vi "Process 1 Page.vi"() -> ()   [LabVIEW 2019]
uses:
  <vilib>/NI/Current Value Table/Type Defs/Single Tag.ctl
  <vilib>/NI/Current Value Table/Type Defs/Data Types.ctl
  <vilib>/NI/STM/TCP/Read Meta Data (TCP Ref).vi
  <vilib>/NI/STM/TCP/Get Connection Reference (TCP).vi
  <vilib>/NI/AMC/Read Termination Message.vi
  <vilib>/NI/AMC/Create Single Message.vi
  <vilib>/NI/AMC/Update Message Routing Info.vi
  <vilib>/NI/STM/TCP/Read Meta Data (TCP Clst).vi
  <vilib>/NI/AMC/Globals.vi
  <vilib>/NI/STM/TCP/Write Message (TCP).vi
  <vilib>/NI/AMC/Send Message.vi
  <vilib>/NI/AMC/AMC.lvlib
  <vilib>/NI/STM/NI STM.lvlib
  <vilib>/NI/Current Value Table/Current Value Table.lvlib
panel:
  out "Boolean 5":bool
  out "Pressure (kPa)":dbl(knob) scale=0.0..150.0
  out "RPM":dbl(knob) scale=0.0..3500.0
  out "DI Flow Rate":dbl(knob) scale=0.0..75.0
  in  "Oxide grams to Add 1":dbl=2.0 caption="Oxide grams to Add" min=-1000.0 max=1000.0 step=0.1
  in  "Dose Extra Oxide 1":bool caption="Dose Extra Oxide"
  in  "Flow to Oxide 1":dbl=2.0 caption="Flow to Oxide" min=2.0 max=12.0 step=0.1
  in  "Enable Oxide System 1":bool caption="Enable Oxide System"
  out "SG":dbl format="%.4g"
  in  "Bath SG":dbl=1.8 min=0.9 max=1.8 step=0.0025 format="%.4g"
  out "Recirc Elbow":bool
  out "Di Add Pipe":bool
  out "Di Water Elbow":bool
  out "Liters DI Added 1":dbl caption="Liters DI Added" format="%.1f"
  in  "T Setpoint 1":dbl=15.0 caption="T Setpoint" min=15.0 max=28.0 step=0.5
  in  "Enable T Control 1":bool caption="Enable T Control"
  in  "DI Add Volume 1":dbl caption="DI Add Volume" min=0.0 max=500.0 step=0.25
  in  "Add DI water 1":bool caption="Add DI Water"
  in  "Drain System to Tree 1":bool caption="Drain System to Tree"
  in  "Enable Main Pump":bool
  out "FlowToOxSys 1":dbl(slide) caption="Flow To Oxide Sys" scale=0.0..12.0 scale format="%.1f"
  out "Oxide Pump":bool
  out "Chilled Water Injection 1":u8(slide) caption="Chilled Water Injection" scale=0.0..100.0
  out "Tempered Water Injection 1":u8(slide) caption="Tempered Water Injection" scale=0.0..100.0
  out "Process 1 Supply":bool
  out "Sump Return":bool
  out "PipeFromPmp":bool
  out "Plating Tanks In Use South PE":bool
  out "Oxide Left To Dose":dbl format="%#.1f"
  out "OxideDose Indicate 1":bool caption="Oxide Dosing"
  out "T °C 1":dbl(slide) caption="T °C" scale=0.0..30.0
  out "Proc4MainPumpInd 2":bool
  out "Tank 1":dbl(slide) caption="Tank" scale=0.0..1000.0
  out "Run Enabled":bool
  in  "Dosing":bool
  in  "Mixing Tank":bool
  in  "Process 3":bool
  in  "Process 2":bool
  in  "Process 1":bool
  out "status":string
  in  "Home Btn":bool
  in  "Facilities Btn":bool
  # "T 341"
  # "@"
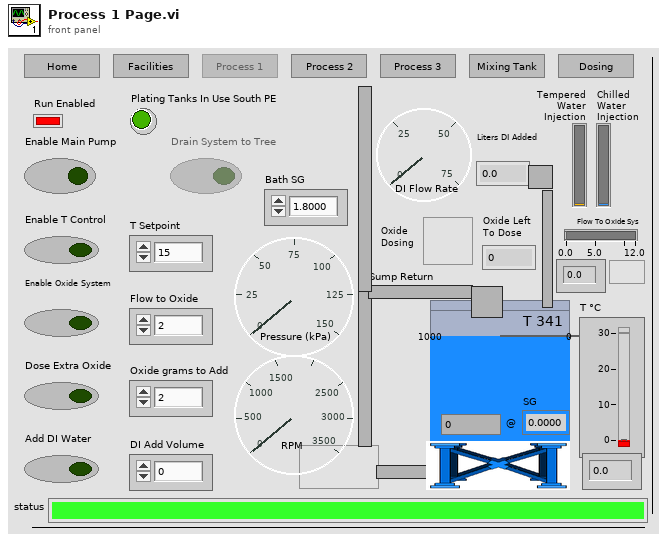
[diagram p1: front panel]
types:
  T1 = typedef "Current Value Table.lvlib/Single Tag.ctl" = cluster{"Data Type":T2, "Name":string, "Value":string, "Description":string}
  T2 = typedef "Current Value Table.lvlib/Data Types.ctl" = enum16{"Double", "Single", "I64", "I32", "I16", "I8", "U64", "U32", "U16", "U8", "String", "Boolean", "Array of U8", "Array of U16", "Array of U32", "Array of U64", "Array of I64", "Array of I32", "Array of I16", "Array of I8", "Array of Double", "Array of Single", "Array of Boolean", "Array of String"}
  T3 = typedef "AMC.lvlib/Message Queue.ctl" = refnum<queue>
  T4 = typedef "NI STM.lvlib/TCP Connection Info.ctl" = cluster{"connection ID":refnum<k5>, "meta data":T5[]}
  T5 = typedef "NI STM.lvlib/MetaDataElement.ctl" = string
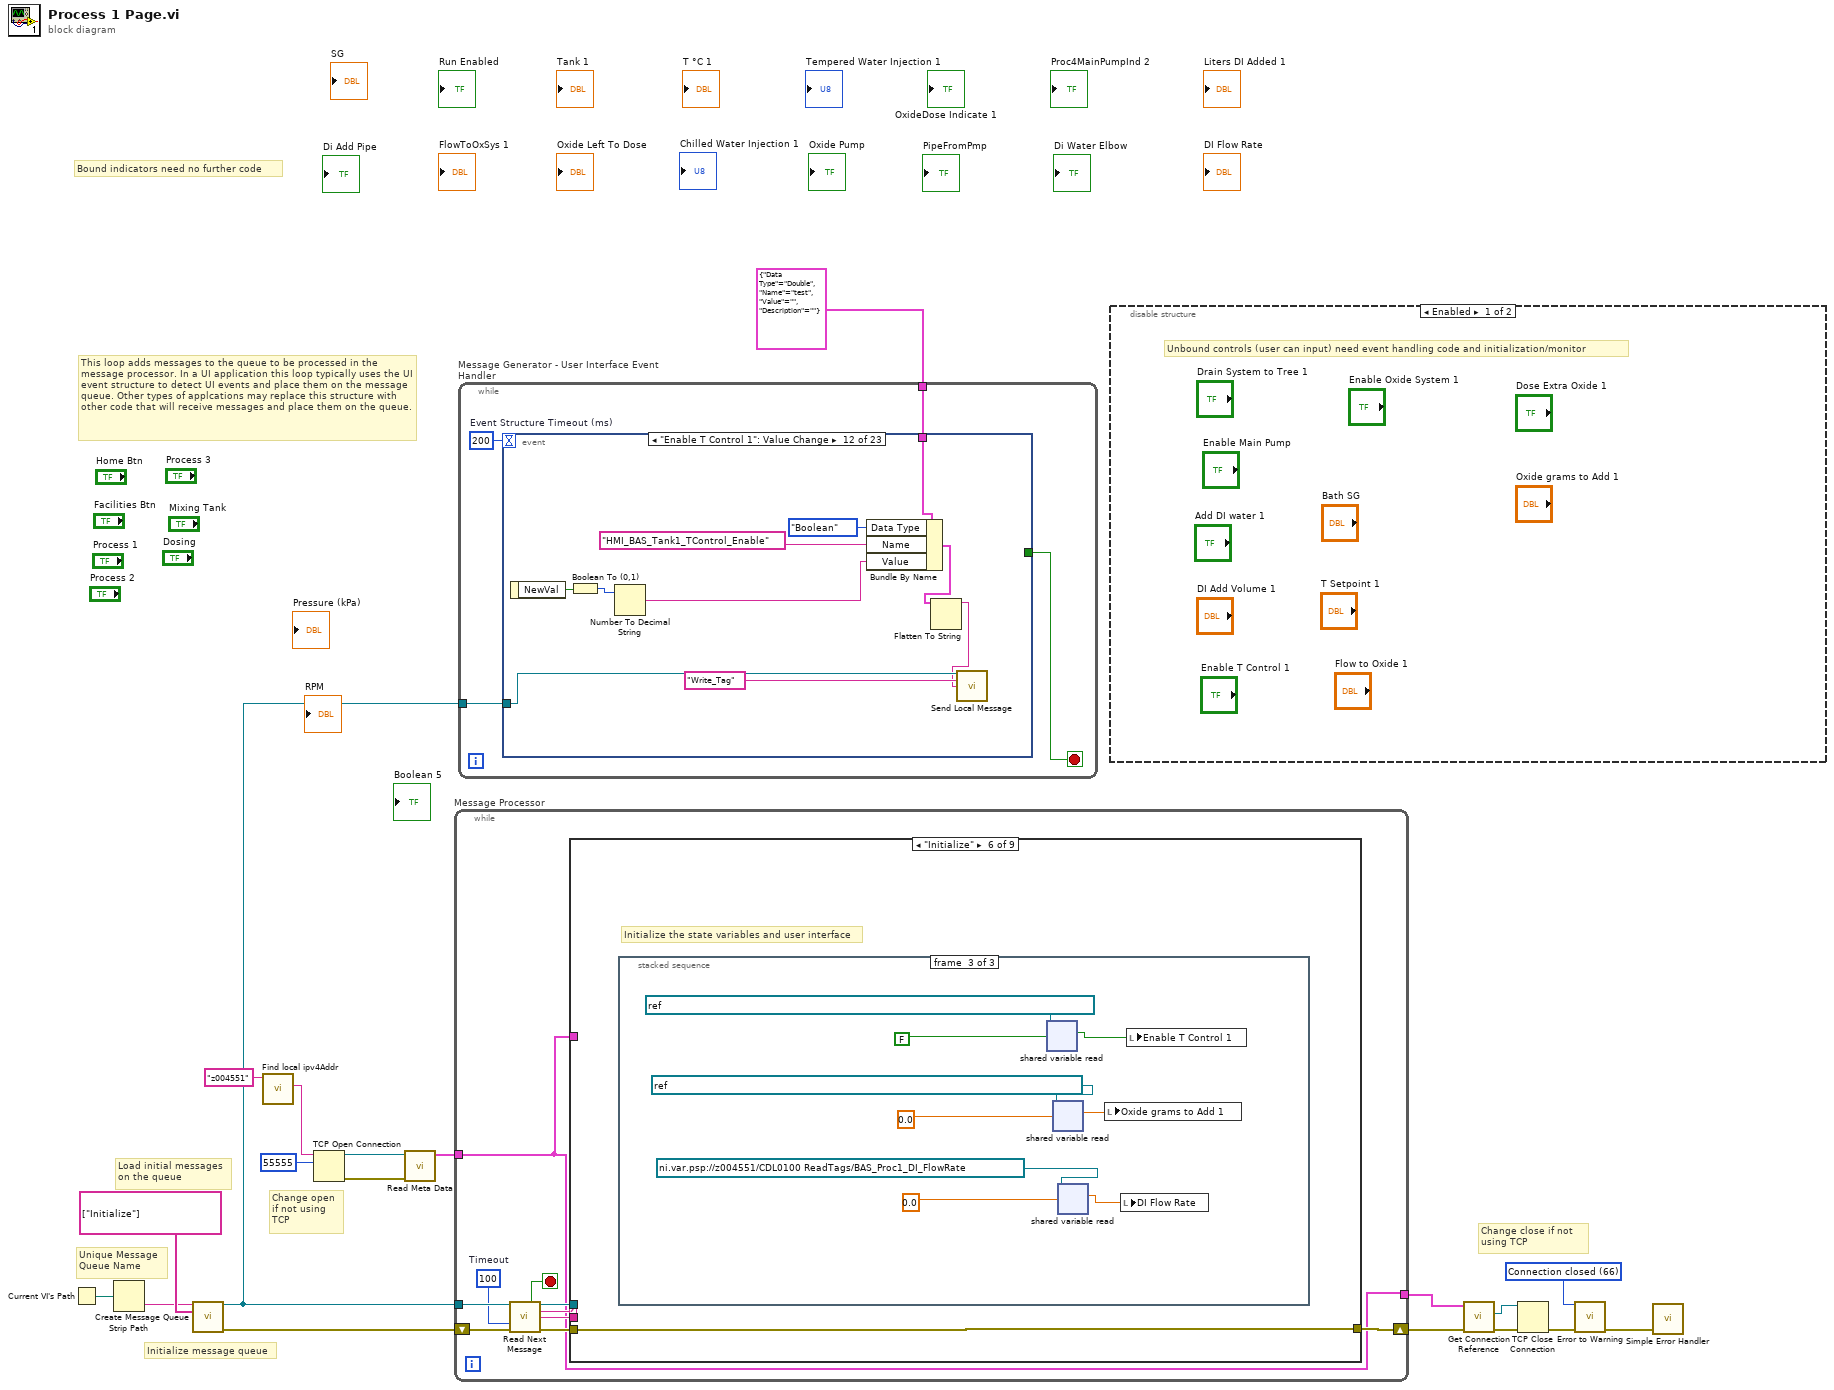
[diagram p0: block diagram]
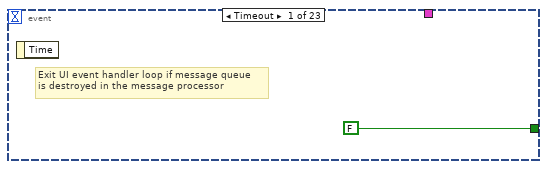
[diagram p3: hidden frame]
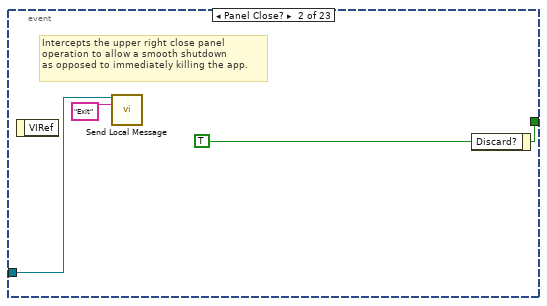
[diagram p4: hidden frame]
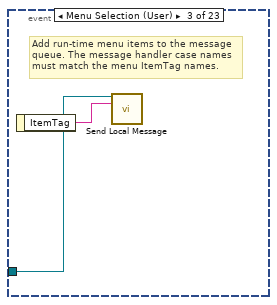
[diagram p5: hidden frame]
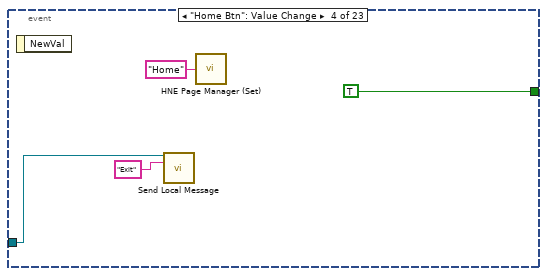
[diagram p6: hidden frame]
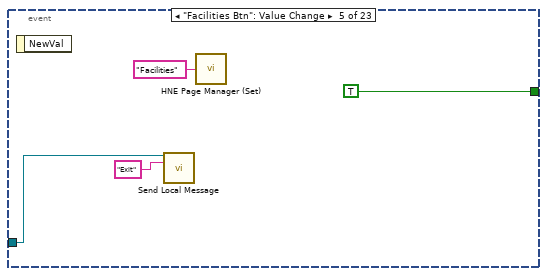
[diagram p7: hidden frame]
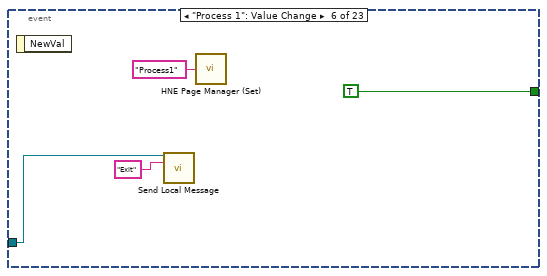
[diagram p8: hidden frame]
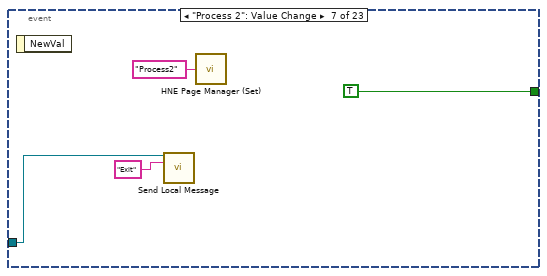
[diagram p9: hidden frame]
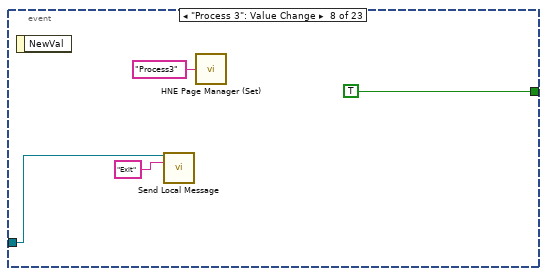
[diagram p10: hidden frame]
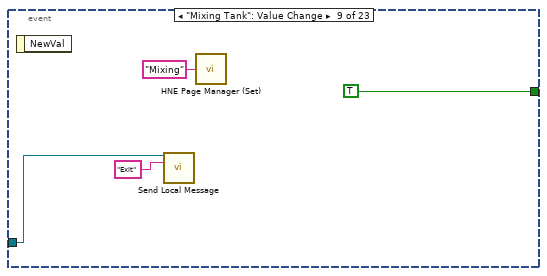
[diagram p11: hidden frame]
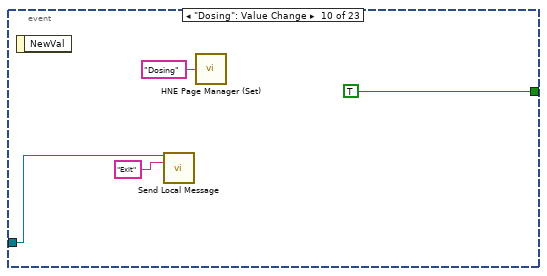
[diagram p12: hidden frame]
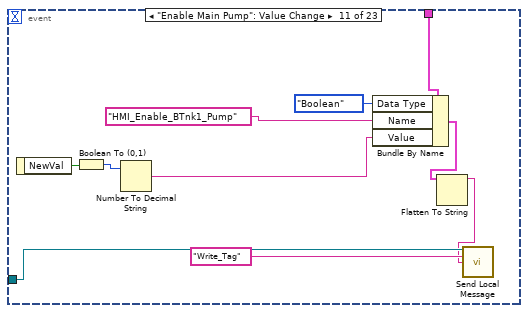
[diagram p13: hidden frame]
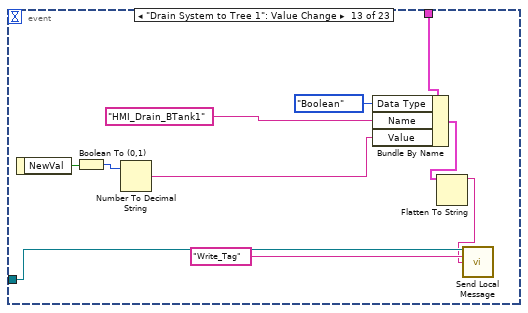
[diagram p14: hidden frame]
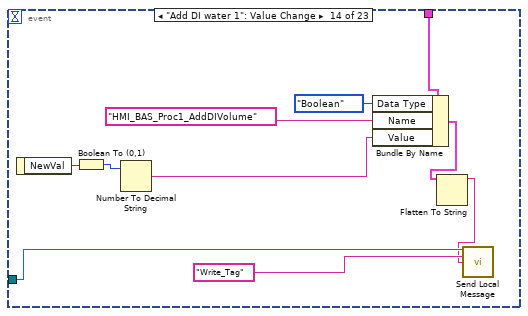
[diagram p15: hidden frame]
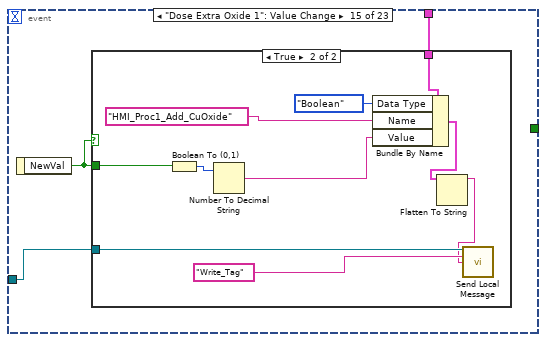
[diagram p16: hidden frame]
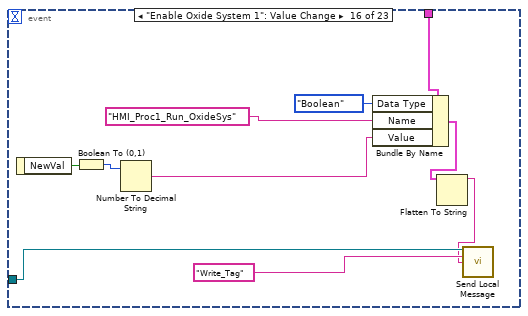
[diagram p18: hidden frame]
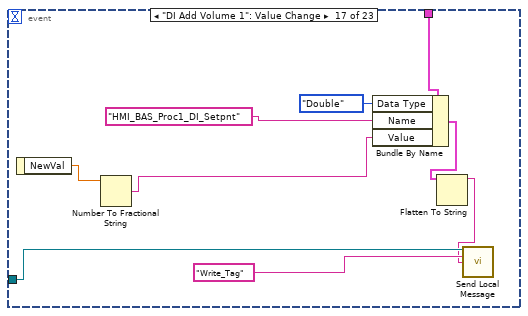
[diagram p19: hidden frame]
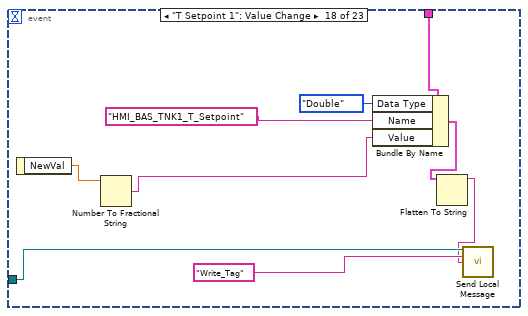
[diagram p20: hidden frame]
diagram:
  w8 = 66 items=["No Error", "Argument Error", "Memory Full", "Out of Zone", "End of File", "File Already Open", "Generic File IO Error", "File Not Found", "File Permission Error", "Disk Full", "Duplicate Path", "Too Many Files Open", "Not Enabled", "Resource File Not Found", "Cannot Add Resource", "Resource Not Found", "Image Not Found", "Image Memory Error", "Pen Does Not Exist", "Config Bad Type", "Config Token Not Found", "Config Parse Error", "Config Memory Error", "Bad External Code Format", "Bad External Code Offset", "External Code Not Present", "Null Window", "Destroy Window Mixup", "Null Menu", "Print Aborted", "Bad Print Record", "Print Driver Error", "Windows Error During Print", "Memory Error During Print", "Print Dialog Error", "Generic Print Error", "Invalid Device Refnum", "Device Not Found", "Device Parameter Error", "Device Unit Error", "Can't Open Device", "Device Call Aborted", "Generic Error", "Cancelled By User", "Object ID Too Low", "Object ID Too High", "Object Not In Heap", "Unknown Heap", "Bad DefProc ID", "DefProc Not In Table", "Message Out Of Range", "Null Method", "Unknown Message", "Manager Call Not Supported", "Bad address", "Connection In progress", "Connection timed out", "Connection is already in progress", "Network attribute not supported", "Network error", "Address in use", "System out of memory", "Connection aborted", "Connection refused", "Connection is not connected", "Connection is already connected", "Connection closed", "Initialize error (interapplication manager)", "Bad occurrence", "Wait on unbound occurrence handler", "Occurrence queue overflow", "Bad path", "Semaphore not signaled", "Unrecognized type (interapplication manager)"] ("1st Error to Convert")
  # "Bound indicators need no further code"
  # "Change close if not using TCP"
  # "Change open if not using TCP"
  # "This loop adds messages to the queue to be processed in the message processor. In a UI application this loop typically uses the UI event structure to detect UI events and place them on the message queue. Other types of applcations may replace this structure with other code that will receive messages and place them on the queue."
  # "Initialize message queue"
  # "Unique Message\nQueue Name"
  # "Load initial messages\non the queue"
  n1 = Current VI's Path() -> (path=w15:path)
  n2 = Strip Path(path=w15) -> (name=w18:string)  [unwired: 1 out]
  n3 = call <vilib>:"Create Message Queue.vi"("message queue name"=w18, "initial message names"=string[] ["Initialize"]) -> ("message queue out"=w17:T3, "error out"=w16:errorcluster)  [unwired: 12 in]
  n4 = call "Find local ipv4Addr.vi"("MachineToFind"="z004551") -> ("name"=w11:string)  [unwired: 9 in, 1 out]
  n5 = TCP Open Connection(address=w11, remote port or service name=u16 55555 ("remote port")) -> (connection ID=w13:refnum<k5>, error out=w12:errorcluster)  [unwired: 1 in, 2 out]
  n6 = call-poly <vilib>:"Read Meta Data.vi"("error in"=w12, "connection ID"=w13) -> ("connection info out"=w3:T4)  [unwired: 7 in, 2 out]
  n7 = while "Message Processor" {
    shift-left: w16 -> [w25]
    shift-right: [w29] -> w4
    tunnel: w17 -> [w26]
    tunnel: [w20] -> w2
    tunnel: w3 -> [w20]
    stop <- w28 stop-if-true
    w21 = 100  # Timeout
    n8 = call <vilib>:"Read Next Message.vi"("message queue in"=w26, "timeout (1 ms)"=w21, "error in"=w25) -> ("exit process?"=w28:bool, "message queue out"=w27:T3, "message name"=w23:string, "message value"=w22:string, "error out"=w24:errorcluster)  [unwired: 5 in, 3 out]
    n9 = case shown="\"Initialize\"" w23 {
      selector: w23 -> [_ _ w69 _ _ _ _ _ _]
      tunnel: w27 -> [_ _ _ _ _ _ w109 _ _]
      tunnel: w24 -> [w30 w32 w70 w71 w73 w74 w110 w112 w114]
      tunnel: [w30 w32 w70 errorcluster {"status"=FALSE, "code"=0, "source"=""} ("error out") w73 w74 w108 w112 w113] -> w29
      tunnel: w22 -> [_ _ _ _ _ _ _ _ w115]
      tunnel: w20 -> [_ _ _ _ _ _ _ _ w116]
      frame "---------- Framework Operations ----------" {
        # "Dummy case to add a seperator in the Case Structure menu"
      }
      frame "", "Idle" {
        # "Idle Case - this case is called after a Timeout on the Get Next Message from Queue VI, if no new messages are present on the queue. This case can be used for housekeeping tasks such as updating the UI."
        n10 = stacked-sequence {
          frame #0 {
            # "Other HMI changed state - align"
            n11 = shared-variable-read(refnum<k21> "ni.var.psp://z004551/CDL0100 ReadWriteTags/HMI_Enable_BTnk1_Pump" ("shared variable refnum in"), FALSE ("data type")) -> (w33:bool)  [unwired: 1 in, 3 out]
            n12 = shared-variable-read(refnum<k21> "ni.var.psp://z004551/CDL0100 ReadWriteTags/HMI_Tank2_Enable" ("shared variable refnum in"), FALSE) -> (w41:bool)  [unwired: 1 in, 3 out]
            n13 = shared-variable-read(refnum<k21> "ni.var.psp://z004551/CDL0100 ReadWriteTags/HMI_Tank1_Enable" ("shared variable refnum in"), FALSE) -> (w36:bool)  [unwired: 1 in, 3 out]
            n14 = Or(x=w36, y=w41) -> (x .or. y?=→"Plating Tanks In Use South PE":bool)
            n15 = call <userlib>:"Boolean Trigger__ogtk.vi"("Boolean Input"=w33) -> ("Rising Edge"=w39:bool, "Falling Edge"=w38:bool)  [unwired: 1 in]
            n16 = Or(x=w39, y=w38) -> (x .or. y?=w37:bool)
            n17 = case shown="True" w37 {
              tunnel: w33 -> [_ w46]
              frame False {
              }
              frame True {
                n18 = local write "Enable Main Pump"(w46) -> ()
              }
            }
          }
          frame #1 {
            n19 = shared-variable-read(refnum<k21> "ni.var.psp://z004551/CDL0100 ReadTags/IO_Bas_Tnk1_3Way_At_Open" ("shared variable refnum in"), FALSE) -> (w49:bool)  [unwired: 1 in, 3 out]
            n20 = shared-variable-read(refnum<k21> "ni.var.psp://z004551/CDL0100 ReadTags/IO_Bas_Tnk1_3Way_At_Recirc" ("shared variable refnum in"), FALSE) -> (w48:bool)  [unwired: 1 in, 3 out]
            n21 = shared-variable-read(refnum<k21> "ni.var.psp://z004551/CDL0100 ReadTags/IO_Bas_Tnk1_3Way_At_Closed" ("shared variable refnum in"), FALSE) -> (w51:bool)  [unwired: 1 in, 3 out]
            n22 = Or(x=w51, y=w49) -> (x .or. y?=→"Process 1 Supply":bool)
            n23 = Or(x=w49, y=w48) -> (x .or. y?=→"Sump Return" →"Recirc Elbow":bool)
          }
          frame #2 {
            n24 = shared-variable-read(refnum<k21> "ni.var.psp://z004551/CDL0100 ReadWriteTags/HMI_BAS_Proc1_AddDIVolume" ("shared variable refnum in"), FALSE) -> (w59:bool)  [unwired: 1 in, 3 out]
            n25 = call <userlib>:"Boolean Trigger__ogtk.vi"("Boolean Input"=w59) -> ("Falling Edge"=w58:bool)  [unwired: 1 in, 1 out]
            n26 = case shown="True" w58 {
              frame False {
              }
              frame True {
                n27 = local write "Add DI water 1"(FALSE) -> ()
              }
            }
          }
          frame #3 {
            n28 = control-ref of="Enable Main Pump"() -> (w63:refnum<vi>)
            n29 = control-ref of="Drain System to Tree 1"() -> (w65:refnum<vi>)
            n30 = call "GrayOutButtonFromPSPVar.vi"("shared variable refnum in"=refnum<k21> "ni.var.psp://z004551/CDL0100 ReadWriteTags/HMI_Drain_BTank1", "Boolean in"=w63) -> ()  [unwired: 10 in]
            n31 = call "GrayOutButtonFromPSPVar.vi"("shared variable refnum in"=refnum<k21> "ni.var.psp://z004551/CDL0100 ReadWriteTags/HMI_Enable_BTnk1_Pump", "Boolean in"=w65) -> ()  [unwired: 10 in]
          }
        }
        n32 = control-ref of="status"() -> (w31:refnum<vi>)
        n33 = call <userlib>:"TAE Format Alarm Ticker.vi"("Alarm Ticker Ref"=w31) -> ()  [unwired: 15 in]
      }
      frame "Missing Message Handler", Default {
        # "Call this case if a message is received that is not handled \nby any other case. Typically this is a programming error\nas a result of a typo or unhandled message/missing message handler."
        n34 = Format Into String(format string="DevError: Missing message handler for '%s\" message." ("message"), w69) -> (resulting string=w67:string)  [unwired: 2 in, 1 out]
        n35 = One Button Dialog(message=w67) -> ()  [unwired: 2 out]
      }
      frame "Error" {
        # "General Error Case - this case is called if an error is passed using the error cluster below. Typically most new errors should be handed in each individual case and not passed in the rror cluster. If necessary a custom error handler case should be added and called from other cases."
        n36 = call <vilib>:"Simple Error Handler.vi"("error in (no error)"=w71) -> ()  [unwired: 1 in, 8 out]
      }
      frame "---------- Generic Operations ----------" {
        # "Dummy case to add a seperator in the Case Structure menu"
      }
      frame "Initialize" {
        # "Initialize the state variables and user interface"
        n37 = stacked-sequence {
          frame #0 {
            n38 = shared-variable-read(refnum<k21> "ni.var.psp://z004551/CDL0100 ReadWriteTags/HMI_Drain_BTank1" ("shared variable refnum in"), FALSE) -> (w81:bool)  [unwired: 1 in, 3 out]
            n39 = shared-variable-read(refnum<k21> "ni.var.psp://z004551/CDL0100 ReadWriteTags/HMI_BAS_Proc1_AddDIVolume" ("shared variable refnum in"), FALSE) -> (w78:bool)  [unwired: 1 in, 3 out]
            n40 = shared-variable-read(refnum<k21> "ni.var.psp://z004551/CDL0100 ReadWriteTags/HMI_Enable_BTnk1_Pump" ("shared variable refnum in"), FALSE) -> (w84:bool)  [unwired: 1 in, 3 out]
            n41 = shared-variable-read(refnum<k21> "ni.var.psp://z004551/CDL0100 ReadWriteTags/HMI_BAS_Proc1_DI_Setpnt" ("shared variable refnum in"), 0.0) -> (w75:dbl)  [unwired: 1 in, 3 out]
            n42 = local write "Drain System to Tree 1"(w81) -> ()
            n43 = local write "Add DI water 1"(w78) -> ()
            n44 = local write "Enable Main Pump"(w84) -> ()
            n45 = local write "DI Add Volume 1"(w75) -> ()
          }
          frame #1 {
            n46 = shared-variable-read(refnum<k21> "ni.var.psp://z004551/CDL0100 ReadWriteTags/HMI_Proc1_Run_OxideSys" ("shared variable refnum in"), FALSE) -> (w87:bool)  [unwired: 1 in, 3 out]
            n47 = shared-variable-read(refnum<k21> "ni.var.psp://z004551/CDL0100 ReadWriteTags/HMI_Proc1_OxFlow_SetPnt" ("shared variable refnum in"), 0.0) -> (w90:dbl)  [unwired: 1 in, 3 out]
            n48 = shared-variable-read(refnum<k21> "ni.var.psp://z004551/CDL0100 ReadWriteTags/HMI_BAS_TNK1_T_Setpoint" ("shared variable refnum in"), 0.0) -> (w93:dbl)  [unwired: 1 in, 3 out]
            n49 = shared-variable-read(refnum<k21> "ni.var.psp://z004551/CDL0100 ReadWriteTags/HMI_BAS_Proc1_Tank_SG" ("shared variable refnum in"), 0.0) -> (w96:dbl)  [unwired: 1 in, 3 out]
            n50 = local write "Enable Oxide System 1"(w87) -> ()
            n51 = local write "T Setpoint 1"(w93) -> ()
            n52 = local write "Flow to Oxide 1"(w90) -> ()
            n53 = local write "Bath SG"(w96) -> ()
          }
          frame #2 {
            n54 = shared-variable-read(refnum<k21> "ni.var.psp://z004551/CDL0100 ReadWriteTags/HMI_BAS_Tank1_TControl_Enable" ("shared variable refnum in"), FALSE) -> (w105:bool)  [unwired: 1 in, 3 out]
            n55 = shared-variable-read(refnum<k21> "ni.var.psp://z004551/CDL0100 ReadWriteTags/HMI_Proc1_CuOxideAddAmnt" ("shared variable refnum in"), 0.0) -> (w102:dbl)  [unwired: 1 in, 3 out]
            n56 = shared-variable-read(refnum<k21> "ni.var.psp://z004551/CDL0100 ReadTags/BAS_Proc1_DI_FlowRate" ("shared variable refnum in"), 0.0) -> (w99:dbl)  [unwired: 1 in, 3 out]
            n57 = local write "Oxide grams to Add 1"(w102) -> ()
            n58 = local write "DI Flow Rate"(w99) -> ()
            n59 = local write "Enable T Control 1"(w105) -> ()
          }
        }
      }
      frame "Exit" {
        # "Destroy message queue >> this will halt the UI event handler loop"
        # "Stop the VI\n>> Perform any cleanup tasks in this message case.\n>> Clear display before closing."
        n60 = call <vilib>:"Destroy Message Queue.vi"("message queue in"=w109, "error in"=w110) -> ("error out"=w108:errorcluster)  [unwired: 11 in, 2 out]
        n61 = local write "status"("" ("Status")) -> ()
      }
      frame "---------- Application Operations ----------" {
        # "Dummy case to add a seperator in the Case Structure menu"
      }
      frame "Write_Tag" {
        n62 = call-poly <vilib>:"Write Message.vi"("error in"=w114, "data"=w115, "name"="WriteTag", "connection info in"=w116) -> ("error out"=w113:errorcluster)  [unwired: 6 in, 1 out]
      }
    }
  }
  n63 = while "Message Generator - User Interface Event Handler" {
    tunnel: w17 -> [w119]
    tunnel: T1 {"Data Type"=enum."Double", "Name"="test", "Value"="", "Description"=""} ("Tag") -> [w118]
    stop <- w120 stop-if-true
    w121 = 200  # Event Structure Timeout (ms)
    n64 = event shown="[11] \"Enable T Control 1\": Value Change" {
      selector: _ -> [_ _ _ _ _ _ _ _ _ _ _ _ _ _ _ _ _ _ _ _ _ _ _]
      dyn-events: _ -> [_ _ _ _ _ _ _ _ _ _ _ _ _ _ _ _ _ _ _ _ _ _ _]
      timeout: w121 -> [_ _ _ _ _ _ _ _ _ _ _ _ _ _ _ _ _ _ _ _ _ _ _]
      tunnel: [FALSE ("Discard?") w125 _ TRUE ("Discard?") TRUE ("Discard?") TRUE ("Discard?") TRUE ("Discard?") TRUE ("Discard?") TRUE ("Discard?") TRUE ("Discard?") _ _ _ _ _ _ _ _ _ _ _ _ _] -> w120
      tunnel: w119 -> [_ w123 w126 w128 w132 w136 w140 w144 w148 w152 w158 w168 w178 w188 w197 w211 w223 w232 w241 w250 w259 _ _]
      tunnel: w118 -> [_ _ _ _ _ _ _ _ _ _ w163 w173 w183 w193 w198 w216 w227 w236 w245 w254 w263 _ _]
      event Timeout {
        # "Exit UI event handler loop if message queue\nis destroyed in the message processor"
        n65 = event-data() -> ()  [unwired: 2 out]
      }
      event Panel Close? {
        w125 = TRUE ("Discard?")
        # "Intercepts the upper right close panel\noperation to allow a smooth shutdown\nas opposed to immediately killing the app."
        n66 = event-data() -> ()  [unwired: 2 out]
        n67 = call <vilib>:"Send Local Message.vi"("message queue in"=w123, "message name"="Exit") -> ()  [unwired: 11 in, 3 out]
        n68 = event-data("Discard?"=w125) -> ()  [unwired: 1 in, 1 out]
      }
      event Menu Selection (User) {
        # "Add run-time menu items to the message\nqueue. The message handler case names must match the menu ItemTag names."
        n69 = event-data() -> ("ItemTag"=w127:string)  [unwired: 1 out]
        n70 = call <vilib>:"Send Local Message.vi"("message queue in"=w126, "message name"=w127) -> ()  [unwired: 11 in, 3 out]
      }
      event "Home Btn": Value Change {
        n71 = event-data() -> ()  [unwired: 2 out]
        n72 = call <vilib>:"Send Local Message.vi"("message queue in"=w128, "message name"="Exit") -> ()  [unwired: 11 in, 3 out]
        n73 = call <userlib>:"HNE Page Manager (Set).vi"("Next Page"="Home") -> ()  [unwired: 4 in, 1 out]
      }
      event "Facilities Btn": Value Change {
        n74 = event-data() -> ()  [unwired: 2 out]
        n75 = call <vilib>:"Send Local Message.vi"("message queue in"=w132, "message name"="Exit") -> ()  [unwired: 11 in, 3 out]
        n76 = call <userlib>:"HNE Page Manager (Set).vi"("Next Page"="Facilities") -> ()  [unwired: 4 in, 1 out]
      }
      event "Process 1": Value Change {
        n77 = event-data() -> ()  [unwired: 2 out]
        n78 = call <vilib>:"Send Local Message.vi"("message queue in"=w136, "message name"="Exit") -> ()  [unwired: 11 in, 3 out]
        n79 = call <userlib>:"HNE Page Manager (Set).vi"("Next Page"="Process1") -> ()  [unwired: 4 in, 1 out]
      }
      event "Process 2": Value Change {
        n80 = event-data() -> ()  [unwired: 2 out]
        n81 = call <vilib>:"Send Local Message.vi"("message queue in"=w140, "message name"="Exit") -> ()  [unwired: 11 in, 3 out]
        n82 = call <userlib>:"HNE Page Manager (Set).vi"("Next Page"="Process2") -> ()  [unwired: 4 in, 1 out]
      }
      event "Process 3": Value Change {
        n83 = event-data() -> ()  [unwired: 2 out]
        n84 = call <vilib>:"Send Local Message.vi"("message queue in"=w144, "message name"="Exit") -> ()  [unwired: 11 in, 3 out]
        n85 = call <userlib>:"HNE Page Manager (Set).vi"("Next Page"="Process3") -> ()  [unwired: 4 in, 1 out]
      }
      event "Mixing Tank": Value Change {
        n86 = event-data() -> ()  [unwired: 2 out]
        n87 = call <vilib>:"Send Local Message.vi"("message queue in"=w148, "message name"="Exit") -> ()  [unwired: 11 in, 3 out]
        n88 = call <userlib>:"HNE Page Manager (Set).vi"("Next Page"="Mixing") -> ()  [unwired: 4 in, 1 out]
      }
      event "Dosing": Value Change {
        n89 = event-data() -> ()  [unwired: 2 out]
        n90 = call <vilib>:"Send Local Message.vi"("message queue in"=w152, "message name"="Exit") -> ()  [unwired: 11 in, 3 out]
        n91 = call <userlib>:"HNE Page Manager (Set).vi"("Next Page"="Dosing") -> ()  [unwired: 4 in, 1 out]
      }
      event "Enable Main Pump": Value Change {
        n92 = event-data() -> ("NewVal"=w165:bool)  [unwired: 1 out]
        n93 = Boolean To (0,1)(Boolean=w165) -> (0, 1=w164:i16)
        n94 = Number To Decimal String(number=w164) -> (decimal integer string=w160:string)  [unwired: 1 in]
        n95 = Bundle By Name(cluster=w163, "Data Type"=Data_Types."Boolean", "Name"="HMI_Enable_BTnk1_Pump", "Value"=w160) -> (w159:T1)
        n96 = Flatten To String(anything=w159) -> (data string=w156:string)  [unwired: 3 in, 2 out]
        n97 = call <vilib>:"Send Local Message.vi"("message queue in"=w158, "message name"="Write_Tag", "message value"=w156) -> ()  [unwired: 10 in, 3 out]
      }
      event "Enable T Control 1": Value Change {
        n98 = event-data() -> ("NewVal"=w175:bool)  [unwired: 1 out]
        n99 = Boolean To (0,1)(Boolean=w175) -> (0, 1=w174:i16)
        n100 = Number To Decimal String(number=w174) -> (decimal integer string=w170:string)  [unwired: 1 in]
        n101 = Bundle By Name(cluster=w173, "Data Type"=Data_Types."Boolean", "Name"="HMI_BAS_Tank1_TControl_Enable", "Value"=w170) -> (w169:T1)
        n102 = Flatten To String(anything=w169) -> (data string=w166:string)  [unwired: 3 in, 2 out]
        n103 = call <vilib>:"Send Local Message.vi"("message queue in"=w168, "message name"="Write_Tag", "message value"=w166) -> ()  [unwired: 10 in, 3 out]
      }
      event "Drain System to Tree 1": Value Change {
        n104 = event-data() -> ("NewVal"=w185:bool)  [unwired: 1 out]
        n105 = Boolean To (0,1)(Boolean=w185) -> (0, 1=w184:i16)
        n106 = Number To Decimal String(number=w184) -> (decimal integer string=w180:string)  [unwired: 1 in]
        n107 = Bundle By Name(cluster=w183, "Data Type"=Data_Types."Boolean", "Name"="HMI_Drain_BTank1", "Value"=w180) -> (w179:T1)
        n108 = Flatten To String(anything=w179) -> (data string=w176:string)  [unwired: 3 in, 2 out]
        n109 = call <vilib>:"Send Local Message.vi"("message queue in"=w178, "message name"="Write_Tag", "message value"=w176) -> ()  [unwired: 10 in, 3 out]
      }
      event "Add DI water 1": Value Change {
        n110 = event-data() -> ("NewVal"=w195:bool)  [unwired: 1 out]
        n111 = Boolean To (0,1)(Boolean=w195) -> (0, 1=w194:i16)
        n112 = Number To Decimal String(number=w194) -> (decimal integer string=w190:string)  [unwired: 1 in]
        n113 = Bundle By Name(cluster=w193, "Data Type"=Data_Types."Boolean", "Name"="HMI_BAS_Proc1_AddDIVolume", "Value"=w190) -> (w189:T1)
        n114 = Flatten To String(anything=w189) -> (data string=w186:string)  [unwired: 3 in, 2 out]
        n115 = call <vilib>:"Send Local Message.vi"("message queue in"=w188, "message name"="Write_Tag", "message value"=w186) -> ()  [unwired: 10 in, 3 out]
      }
      event "Dose Extra Oxide 1": Value Change {
        n116 = event-data() -> ("NewVal"=w196:bool)  [unwired: 1 out]
        n117 = case shown="True" w196 {
          tunnel: w196 -> [_ w208]
          tunnel: w198 -> [_ w206]
          tunnel: w197 -> [_ w201]
          frame False {
          }
          frame True {
            n118 = Boolean To (0,1)(Boolean=w208) -> (0, 1=w207:i16)
            n119 = Number To Decimal String(number=w207) -> (decimal integer string=w203:string)  [unwired: 1 in]
            n120 = Bundle By Name(cluster=w206, "Data Type"=Data_Types."Boolean", "Name"="HMI_Proc1_Add_CuOxide", "Value"=w203) -> (w202:T1)
            n121 = Flatten To String(anything=w202) -> (data string=w199:string)  [unwired: 3 in, 2 out]
            n122 = call <vilib>:"Send Local Message.vi"("message queue in"=w201, "message name"="Write_Tag", "message value"=w199) -> ()  [unwired: 10 in, 3 out]
          }
        }
      }
      event "Enable Oxide System 1": Value Change {
        n123 = event-data() -> ("NewVal"=w218:bool)  [unwired: 1 out]
        n124 = Boolean To (0,1)(Boolean=w218) -> (0, 1=w217:i16)
        n125 = Number To Decimal String(number=w217) -> (decimal integer string=w213:string)  [unwired: 1 in]
        n126 = Bundle By Name(cluster=w216, "Data Type"=Data_Types."Boolean", "Name"="HMI_Proc1_Run_OxideSys", "Value"=w213) -> (w212:T1)
        n127 = Flatten To String(anything=w212) -> (data string=w209:string)  [unwired: 3 in, 2 out]
        n128 = call <vilib>:"Send Local Message.vi"("message queue in"=w211, "message name"="Write_Tag", "message value"=w209) -> ()  [unwired: 10 in, 3 out]
      }
      event "DI Add Volume 1": Value Change {
        n129 = event-data() -> ("NewVal"=w220:dbl)  [unwired: 1 out]
        n130 = Number To Fractional String(number=w220) -> (F-format string=w219:string)  [unwired: 3 in]
        n131 = Bundle By Name(cluster=w227, "Data Type"=Data_Types."Double", "Name"="HMI_BAS_Proc1_DI_Setpnt", "Value"=w219) -> (w224:T1)
        n132 = Flatten To String(anything=w224) -> (data string=w221:string)  [unwired: 3 in, 2 out]
        n133 = call <vilib>:"Send Local Message.vi"("message queue in"=w223, "message name"="Write_Tag", "message value"=w221) -> ()  [unwired: 10 in, 3 out]
      }
      event "T Setpoint 1": Value Change {
        n134 = event-data() -> ("NewVal"=w229:dbl)  [unwired: 1 out]
        n135 = Number To Fractional String(number=w229) -> (F-format string=w228:string)  [unwired: 3 in]
        n136 = Bundle By Name(cluster=w236, "Data Type"=Data_Types."Double", "Name"="HMI_BAS_TNK1_T_Setpoint", "Value"=w228) -> (w233:T1)
        n137 = Flatten To String(anything=w233) -> (data string=w230:string)  [unwired: 3 in, 2 out]
        n138 = call <vilib>:"Send Local Message.vi"("message queue in"=w232, "message name"="Write_Tag", "message value"=w230) -> ()  [unwired: 10 in, 3 out]
      }
      event "Bath SG": Value Change {
        n139 = event-data() -> ("NewVal"=w238:dbl)  [unwired: 1 out]
        n140 = Number To Fractional String(number=w238) -> (F-format string=w237:string)  [unwired: 3 in]
        n141 = Bundle By Name(cluster=w245, "Data Type"=Data_Types."Double", "Name"="HMI_BAS_Proc1_Tank_SG", "Value"=w237) -> (w242:T1)
        n142 = Flatten To String(anything=w242) -> (data string=w239:string)  [unwired: 3 in, 2 out]
        n143 = call <vilib>:"Send Local Message.vi"("message queue in"=w241, "message name"="Write_Tag", "message value"=w239) -> ()  [unwired: 10 in, 3 out]
      }
      event "Flow to Oxide 1": Value Change {
        n144 = event-data() -> ("NewVal"=w247:dbl)  [unwired: 1 out]
        n145 = Number To Fractional String(number=w247) -> (F-format string=w246:string)  [unwired: 3 in]
        n146 = Bundle By Name(cluster=w254, "Data Type"=Data_Types."Double", "Name"="HMI_Proc1_OxFlow_SetPnt", "Value"=w246) -> (w251:T1)
        n147 = Flatten To String(anything=w251) -> (data string=w248:string)  [unwired: 3 in, 2 out]
        n148 = call <vilib>:"Send Local Message.vi"("message queue in"=w250, "message name"="Write_Tag", "message value"=w248) -> ()  [unwired: 10 in, 3 out]
      }
      event "Oxide grams to Add 1": Value Change {
        n149 = event-data() -> ("NewVal"=w256:dbl)  [unwired: 1 out]
        n150 = Number To Fractional String(number=w256) -> (F-format string=w255:string)  [unwired: 3 in]
        n151 = Bundle By Name(cluster=w263, "Data Type"=Data_Types."Double", "Name"="HMI_Proc1_CuOxideAddAmnt", "Value"=w255) -> (w260:T1)
        n152 = Flatten To String(anything=w260) -> (data string=w257:string)  [unwired: 3 in, 2 out]
        n153 = call <vilib>:"Send Local Message.vi"("message queue in"=w259, "message name"="Write_Tag", "message value"=w257) -> ()  [unwired: 10 in, 3 out]
      }
      event "DI Add Volume 1", "Bath SG", "T Setpoint 1": Mouse Up {
        n154 = event-data() -> ("CtlRef"=w264:refnum<vi>)  [unwired: 8 out]
        n155 = property class="DigNum (strict)"(reference=w264) -> (reference out=w265:refnum<vi>, "Label.Text"=w271:string, "Value"=w270:dbl)  [unwired: 1 in, 1 out]
        n156 = Number To Fractional String(number=w270, precision (6)=i16 1) -> (F-format string=w269:string)  [unwired: 2 in]
        n157 = call <userlib>:"HMI Pop Up Num KP.vi"("String In"=w269, "Message In"=w271) -> ("Canceled"=w267:bool, "String Out"=w266:string)  [unwired: 8 in]
        n158 = case shown="False" w267 {
          tunnel: w266 -> [w273 _]
          tunnel: w265 -> [w274 _]
          frame False {
            n159 = Fract/Exp String To Number(string=w273) -> (number=w272:dbl)  [unwired: 3 in, 1 out]
            n160 = property class="DigNum (strict)"(reference=w274, "Val(Sgnl)"=w272) -> ()  [unwired: 1 in, 2 out]
          }
          frame True {
          }
        }
      }
      event "Flow to Oxide 1", "Oxide grams to Add 1": Mouse Up {
        n161 = event-data() -> ("CtlRef"=w275:refnum<vi>)  [unwired: 8 out]
        n162 = property class="DigNum (strict)"(reference=w275) -> (reference out=w276:refnum<vi>, "Label.Text"=w282:string, "Value"=w281:dbl)  [unwired: 1 in, 1 out]
        n163 = Number To Fractional String(number=w281, precision (6)=i16 1) -> (F-format string=w280:string)  [unwired: 2 in]
        n164 = call <userlib>:"HMI Pop Up Num KP.vi"("String In"=w280, "Message In"=w282) -> ("Canceled"=w278:bool, "String Out"=w277:string)  [unwired: 8 in]
        n165 = case shown="False" w278 {
          tunnel: w277 -> [w284 _]
          tunnel: w276 -> [w285 _]
          frame False {
            n166 = Fract/Exp String To Number(string=w284) -> (number=w283:dbl)  [unwired: 3 in, 1 out]
            n167 = property class="DigNum (strict)"(reference=w285, "Val(Sgnl)"=w283) -> ()  [unwired: 1 in, 2 out]
          }
          frame True {
          }
        }
      }
    }
  }
  n168 = disable-structure shown="Enabled" {
    frame Enabled {
      # "Unbound controls (user can input) need event handling code and initialization/monitor"
    }
    frame Disabled {
    }
  }
  n169 = call-poly <vilib>:"Get Connection Reference.vi"("error in"=w4, "connection info in"=w2) -> ("error out"=w7:errorcluster, "connection ID out"=w6:refnum<k5>)  [unwired: 8 out]
  n170 = TCP Close Connection(connection ID=w6, error in (no error)=w7) -> (error out=w9:errorcluster)  [unwired: 2 out]
  n171 = call <vilib>:"Error to Warning.vi"("1st Error to Convert"=w8, "error in"=w9) -> ("warning out"=w5:errorcluster)  [unwired: 3 in, 10 out]
  n172 = call <vilib>:"Simple Error Handler.vi"("error in (no error)"=w5) -> ()  [unwired: 4 in, 5 out]
